vi "Untitled 5.vi"   [LabVIEW 2013]
types:
  T1 = typedef "WPI_JoystickButtonState.ctl" = cluster{"Button 1":bool, "Button 2":bool, "Button 3":bool, "Button 4":bool, "Button 5":bool, "Button 6":bool, "Button 7":bool, "Button 8":bool, "Button 9":bool, "Button 10":bool, "Button 11":bool, "Button 12":bool}
  T2 = cluster{"Axes":cluster{"X Axis":dbl, "Y Axis":dbl, "Throttle":dbl, "Unused":dbl, "Unused":dbl, "Unused":dbl}, "Buttons":T1}
  T3 = cluster{"X Axis":dbl, "Y Axis":dbl, "Throttle":dbl, "Unused":dbl, "Unused":dbl, "Unused":dbl}
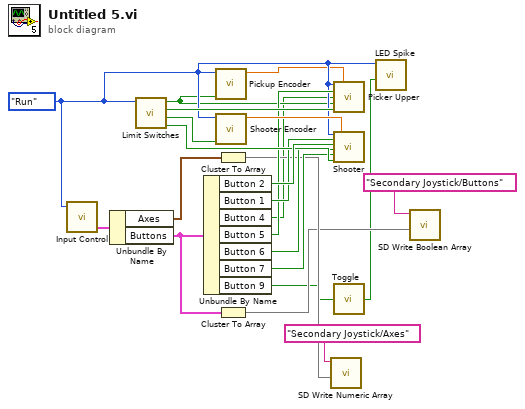
[diagram p0: block diagram]
diagram:
  w12 = enum16{"Open", "Run", "End"}."Run" ("State Control")
  n1 = call "Input Control.vi"("State"=w12) -> ("Secondary Joystick"=w21:T2)  [unwired: 2 in, 2 out]
  n2 = Unbundle By Name(w21) -> ("Axes"=w10:T3, "Buttons"=w7:T1)
  n3 = call "Limit Switches.vi"("State Control"=w12) -> ("Shooter Top"=w19:bool, "Shooter Bottom"=w20:bool, "Picker Upper Bottom"=w18:bool, "Picker Upper Top"=w2:bool)  [unwired: 7 in]
  n4 = Unbundle By Name(w7) -> ("Button 2"=w22:bool, "Button 1"=w17:bool, "Button 4"=w1:bool, "Button 5"=w15:bool, "Button 6"=w14:bool, "Button 7"=w13:bool, "Button 9"=w3:bool)
  n5 = call "Pickup Encoder.vi"("Reset Encoder?"=w2, "State Control"=w12) -> ("Encoder Degrees"=w11:dbl)  [unwired: 2 in, 3 out]
  n6 = call "Shooter Encoder.vi"("Reset Encoder?"=w20, "State Control"=w12) -> ("Encoder Degrees"=w16:dbl)  [unwired: 2 in, 3 out]
  n7 = Cluster To Array(cluster=w10) -> (array=w9:dbl[])
  n8 = Cluster To Array(cluster=w7) -> (array=w6:bool[])
  n9 = call <vilib>:"SD Write Numeric Array.vi"("Numeric Array"=w9, "Name"="Secondary Joystick/Axes") -> ()  [unwired: 8 in, 2 out]
  n10 = call "Picker Upper.vi"("State Control"=w12, "Encoder"=w11, "Up"=w15, "Down"=w1, "Top limit"=w2, "Bottom Limit"=w18) -> ()  [unwired: 8 in, 2 out]
  n11 = call "Shooter.vi"("State Control"=w12, "Manual"=w17, "Return"=w22, "2 ft"=w14, "4 ft"=w13, "Top Limit"=w19, "Encoder"=w16) -> ()  [unwired: 11 in, 2 out]
  n12 = call "Toggle.vi"("Input"=w3) -> ("Latched"=w4:bool)
  n13 = call "LED Spike.vi"("ON/OFF"=w4, "State"=w12) -> ()  [unwired: 10 in]
  n14 = call <vilib>:"SD Write Boolean Array.vi"("Boolean Array"=w6, "Name"="Secondary Joystick/Buttons") -> ()  [unwired: 8 in, 2 out]
